vi "get_data_rate.vi"(8 "error in (no error)":errorcluster, 11 "TrajectoryRK110916Throughput in":refnum<class "TrajectoryRK110916Throughput.lvclass">) -> (0 "error out":errorcluster, 2 "Data rate":u32, 3 "TrajectoryRK110916Throughput out":refnum<class "TrajectoryRK110916Throughput.lvclass">)   [LabVIEW 2010, in "TrajectoryRK110916Throughput.lvclass"]
uses:
  TrajectoryRK110916Throughput.lvclass
  TrajectoryRK110916Throughput.lvclass/TrajectoryRK110916Throughput.ctl
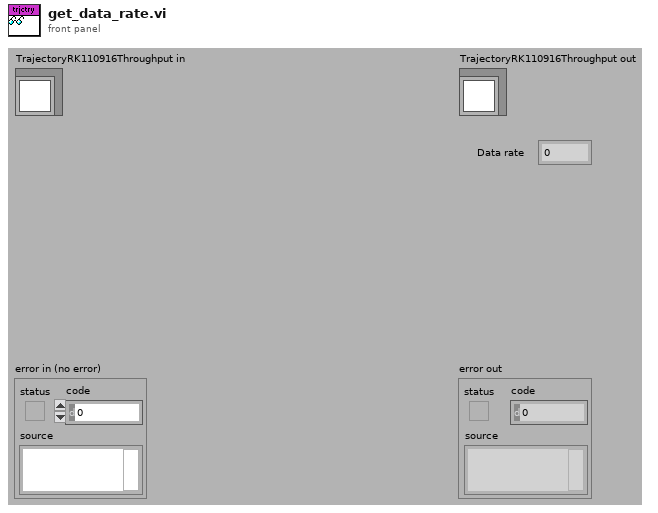
[diagram p1: front panel]
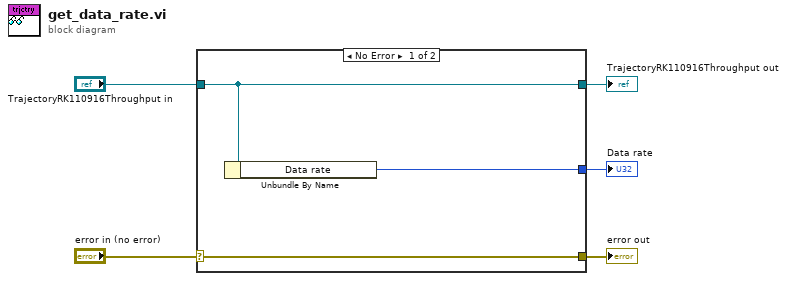
[diagram p0: block diagram]
diagram:
  n1 = case shown="No Error" "error in (no error)" {
    selector: "error in (no error)" -> [w8 w9]
    tunnel: [w8 w9] -> w4
    tunnel: [w7 w10] -> w2
    tunnel: "TrajectoryRK110916Throughput in" -> [w7 w10]
    tunnel: [w6 _] -> w1
    frame No Error {
      n2 = Unbundle By Name(w7) -> ("Data rate"=w6:u32)
    }
    frame Error {
    }
  }
  "error out" <- w4
  "TrajectoryRK110916Throughput out" <- w2
  "Data rate" <- w1
